vi "Q_Driver.vi"(0 "State":string, 2 "Name":string, 5 "States[]":string[](array[string]), 11 "Error In":errorcluster, 13 "Operations":T1) -> (4 "Dequeued Element":string, 15 "Error Out":errorcluster)   [LabVIEW 2020]
doc: "This VI is used as the driver for the queue. It performs the all the operation in queue. Along with Array of elements enqueuing. \nWhen there is a error in error lines this return's the error state by default."
uses:
  Typedef's/Q_Operations.ctl
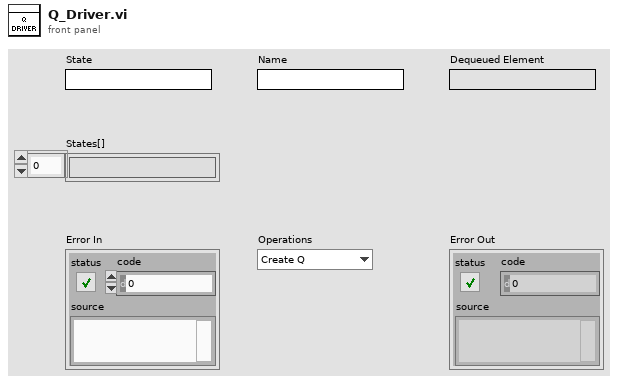
[diagram p1: front panel]
types:
  T1 = typedef "Q_Operations.ctl" = enum16{"Create Q", "Enqueue", "Dequeue", "Enqueue N ele", "Enstack N ele", "Flush Q", "Destroy Q"}
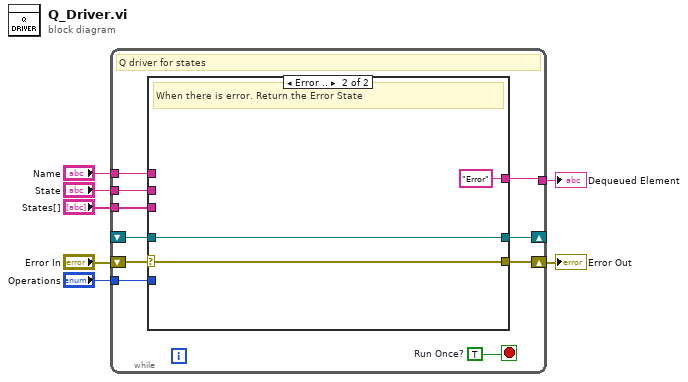
[diagram p0: block diagram]
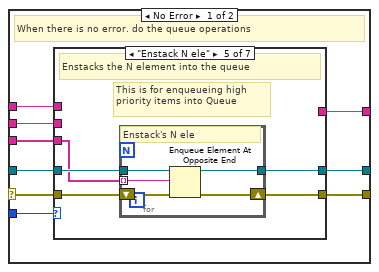
[diagram p2: hidden frame]
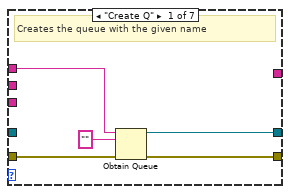
[diagram p3: hidden frame]
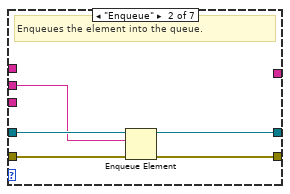
[diagram p4: hidden frame]
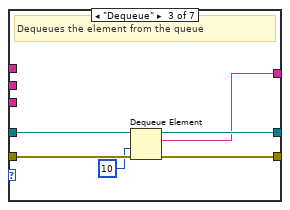
[diagram p5: hidden frame]
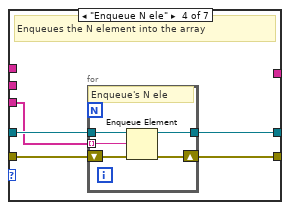
[diagram p6: hidden frame]
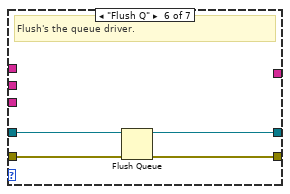
[diagram p7: hidden frame]
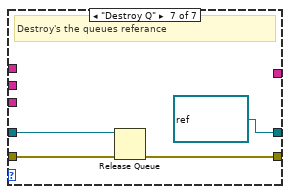
[diagram p8: hidden frame]
diagram:
  n1 = while {
    tunnel: "Operations" -> [w16]
    shift-right: [w14] -> w1
    shift-left: "Error In" -> [w15]
    shift-right: [w13] -> _
    shift-left: _ -> [w12]
    tunnel: "Name" -> [w11]
    tunnel: "State" -> [w10]
    tunnel: "States[]" -> [w9]
    tunnel: [w8] -> w2
    stop <- w17 stop-if-true
    w17 = TRUE  # Run Once?
    # "Q driver for states"
    n2 = case shown="Error .." w15 {
      selector: w15 -> [w25 w73]
      tunnel: w16 -> [w26 _]
      tunnel: [w24 w73] -> w14
      tunnel: [w23 w71] -> w13
      tunnel: w12 -> [w22 w71]
      tunnel: w11 -> [w21 _]
      tunnel: w10 -> [w20 _]
      tunnel: w9 -> [w19 _]
      tunnel: [w18 "Error"] -> w8
      frame No Error {
        # "When there is no error. do the queue operations"
        n3 = case shown="\"Enstack N ele\"" w26 {
          tunnel: w25 -> [w31 w36 w42 w47 w57 w66 w70]
          tunnel: [w30 w35 w41 w46 w56 w65 w69] -> w24
          tunnel: [w29 w33 w40 w44 w55 w64 refnum<queue> refnum ("queue out")] -> w23
          tunnel: w22 -> [_ w34 w39 w45 w54 w63 w68]
          tunnel: w21 -> [w28 _ _ _ _ _ _]
          tunnel: w20 -> [_ w32 _ _ _ _ _]
          tunnel: w19 -> [_ _ _ w43 w53 _ _]
          tunnel: [_ _ w37 _ _ _ _] -> w18
          frame "Create Q" {
            # "Creates the queue with the given name"
            n4 = Obtain Queue(name (unnamed)=w28, element data type="", error in (no error)=w31) -> (queue out=w29:refnum<queue>, error out=w30:errorcluster)  [unwired: 2 in, 1 out]
          }
          frame "Enqueue" {
            # "Enqueues the element into the queue."
            n5 = Enqueue Element(queue=w34, element=w32, error in (no error)=w36) -> (queue out=w33:refnum<queue>, error out=w35:errorcluster)  [unwired: 1 in, 1 out]
          }
          frame "Dequeue" {
            # "Dequeues the element from the queue"
            n6 = Dequeue Element(queue=w39, timeout in ms (-1)=10, error in (no error)=w42) -> (queue out=w40:refnum<queue>, element=w37:string, error out=w41:errorcluster)  [unwired: 1 out]
          }
          frame "Enqueue N ele" {
            # "Enqueues the N element into the array"
            n7 = for {
              tunnel: w45 -> [w50]
              tunnel: [w49] -> w44
              shift-right: [w51] -> w46
              shift-left: w47 -> [w52]
              tunnel: w43 -> [w48] mode=indexing
              # "Enqueue's N ele"
              n8 = Enqueue Element(queue=w50, element=w48, error in (no error)=w52) -> (queue out=w49:refnum<queue>, error out=w51:errorcluster)  [unwired: 1 in, 1 out]
            }
          }
          frame "Enstack N ele" {
            # "This is for enqueueing high priority items into Queue"
            # "Enstacks the N element into the queue"
            n9 = for {
              tunnel: [w60] -> w55
              tunnel: w54 -> [w59]
              shift-right: [w61] -> w56
              shift-left: w57 -> [w62]
              tunnel: w53 -> [w58] mode=indexing
              # "Enstack's N ele"
              n10 = Enqueue Element At Opposite End(queue=w59, element=w58, error in (no error)=w62) -> (queue out=w60:refnum<queue>, error out=w61:errorcluster)  [unwired: 1 in, 1 out]
            }
          }
          frame "Flush Q" {
            # "Flush's the queue driver."
            n11 = Flush Queue(queue=w63, error in (no error)=w66) -> (queue out=w64:refnum<queue>, error out=w65:errorcluster)  [unwired: 1 out]
          }
          frame "Destroy Q" {
            # "Destroy's the queues referance"
            n12 = Release Queue(queue=w68, error in (no error)=w70) -> (error out=w69:errorcluster)  [unwired: 1 in, 2 out]
          }
        }
      }
      frame Error {
        # "When there is error. Return the Error State"
      }
    }
  }
  "Dequeued Element" <- w2
  "Error Out" <- w1
